vi "WF0_Hout_Lout_Verify.vi"(0 "connection ID":refnum<k5>, 1 "time out":i32=40000, 2 "Num_Verify":i32=4, 3 "error out":errorcluster) -> (4 "B-mode(Hout_Lout_Reg)":string[](array[string]), 5 "D-mode(Hout_Lout_Reg)":string[](array[string]), 6 "connection ID 2":refnum<k5>, 7 "time out 2":i32, 8 "Result_RLE":bool, 9 "error out 2":errorcluster caption="error out")   [LabVIEW 2016]
panel:
  out "Same_Hout_Lout_Reg":bool[](array[boolean])
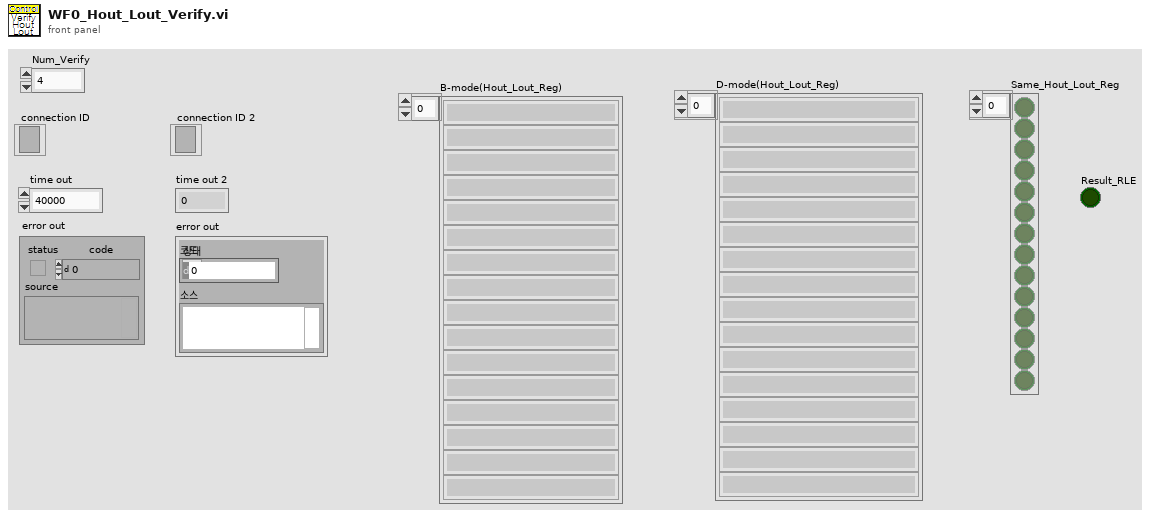
[diagram p1: front panel]
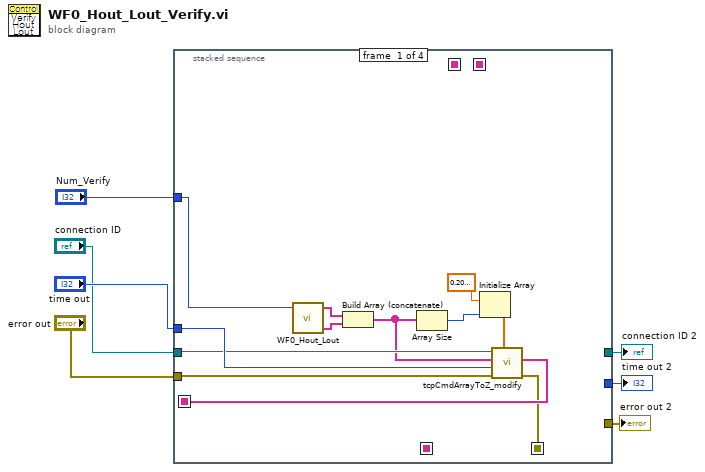
[diagram p0: block diagram]
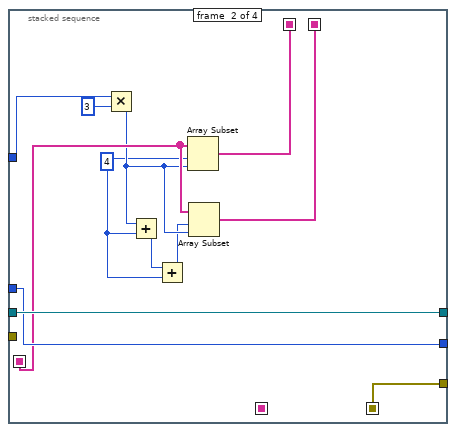
[diagram p2: hidden frame]
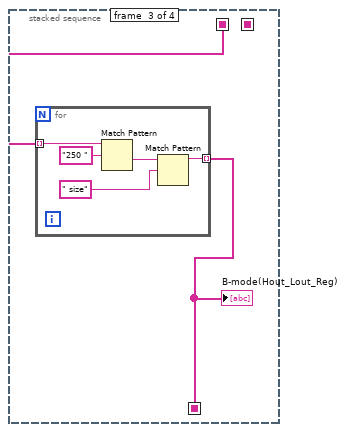
[diagram p3: hidden frame]
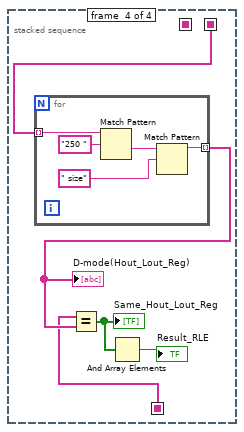
[diagram p4: hidden frame]
diagram:
  n1 = stacked-sequence {
    seq-local: [w9 _ _ _] -> [_ w28 _ _]
    seq-local: [w8 _ _ _] -> [_ w31 _ _]
    seq-local: [_ w21 _ _] -> [_ _ w33 _]
    seq-local: [_ w20 _ _] -> [_ _ _ w43]
    seq-local: [_ _ w32 _] -> [_ _ _ w39]
    tunnel: "time out" -> [w16 w29 _ _]
    tunnel: "connection ID" -> [w15 w30 _ _]
    tunnel: "error out" -> [w14 _ _ _]
    tunnel: "Num_Verify" -> [w13 w27 _ _]
    tunnel: [_ w31 _ _] -> w4
    tunnel: [_ w30 _ _] -> w3
    tunnel: [_ w29 _ _] -> w2
    frame #0 {
      n2 = call "WF0_Hout_Lout.vi"("Num_Read"=w13) -> ("D-mode"=w11:string[], "B-mode"=w12:string[])  [unwired: 3 in]
      n3 = Build Array (concatenate)(w12, w11) -> (w10:string[])
      n4 = Array Size(array=w10) -> (size(s)=w18:i32)
      n5 = Initialize Array(sgl 0.2 ("Element Data"), w18) -> (w17:sgl[])
      n6 = call "tcpCmdArrayToZ_modify.vi"("Delay (sec)"=w17, "error in (no error)"=w14, "Timeout (ms)"=w16, "Command array"=w10, "connection ID in"=w15) -> ("error out"=w8:errorcluster, "Receive array"=w9:string[])  [unwired: 2 in, 3 out]
    }
    frame #1 {
      w23 = 4 ("인덱스")
      n7 = Multiply(x=w27, y=3) -> (x*y=w25:i32)
      n8 = Add(x=w25, y=w23) -> (x+y=w24:i32)
      n9 = Add(x=w24, y=w23) -> (x+y=w22:i32)
      n10 = Array Subset(array=w28, index=w23, length=w25) -> (w21:string[])
      n11 = Array Subset(array=w28, index=w22, length=w25) -> (w20:string[])
    }
    frame #2 {
      n12 = for {
        tunnel: w33 -> [w38] mode=indexing
        tunnel: [w34] -> w32 mode=indexing
        n13 = Match Pattern(string=w38, regular expression="250 " ("정규식")) -> (after substring=w36:string)  [unwired: 1 in, 3 out]
        n14 = Match Pattern(string=w36, regular expression=" size" ("정규식")) -> (before substring=w34:string)  [unwired: 1 in, 3 out]
      }
      "B-mode(Hout_Lout_Reg)" <- w32
    }
    frame #3 {
      n15 = for {
        tunnel: w43 -> [w48] mode=indexing
        tunnel: [w44] -> w40 mode=indexing
        n16 = Match Pattern(string=w48, regular expression="250 " ("정규식")) -> (after substring=w46:string)  [unwired: 1 in, 3 out]
        n17 = Match Pattern(string=w46, regular expression=" size" ("정규식")) -> (before substring=w44:string)  [unwired: 1 in, 3 out]
      }
      "D-mode(Hout_Lout_Reg)" <- w40
      n18 = Equal?(x=w39, y=w40) -> (x = y?=w42:bool[])
      "Same_Hout_Lout_Reg" <- w42
      n19 = And Array Elements(Boolean array=w42) -> (logical AND=→"Result_RLE":bool)
    }
  }
  "error out 2" <- w4
  "connection ID 2" <- w3
  "time out 2" <- w2
